vi "RRI_FFT.vi"() -> ()   [LabVIEW 2023]
uses:
  <vilib>/Analysis/4window.llb/windowTd.ctl
  <vilib>/measure/maspectr.llb/Power Spectrum and PSD Export Mode.ctl
  <vilib>/Analysis/2dsp.llb/Real FFT.vi
  <vilib>/measure/maspectr.llb/FFT Power Spectrum and PSD for 1 Chan (CDB).vi
  <vilib>/Utility/file.llb/Read Delimited Spreadsheet (DBL).vi
  <vilib>/gmath/NI_Gmath.lvlib
  <vilib>/Analysis/NI_AALPro.lvlib
  <vilib>/measure/NI_MAPro.lvlib
panel:
  out "LF/HF":dbl
  out "total power":dbl
  out "HF":dbl
  out "f0":dbl
  out "LF":dbl
  out "magnitude":dbl[](array[numeric])
  out "RRI baseline":cluster{"f0":dbl, "df":dbl, "magnitude":dbl[]}(graph)
  out "Power Spectrum / PSD":cluster{"f0":dbl, "df":dbl, "magnitude":dbl[]} {"magnitude" format="%.2p"; "f0" format="%0.2p"; "df" format="%0.2p"}
  out "baseline RRI inter":cluster{"xi used":dbl[], "yi":dbl[]}[](graph)
  out "RRI baseline 2":dbl[](graph)
  out "CW_baseline_index":dbl[](array[numeric])
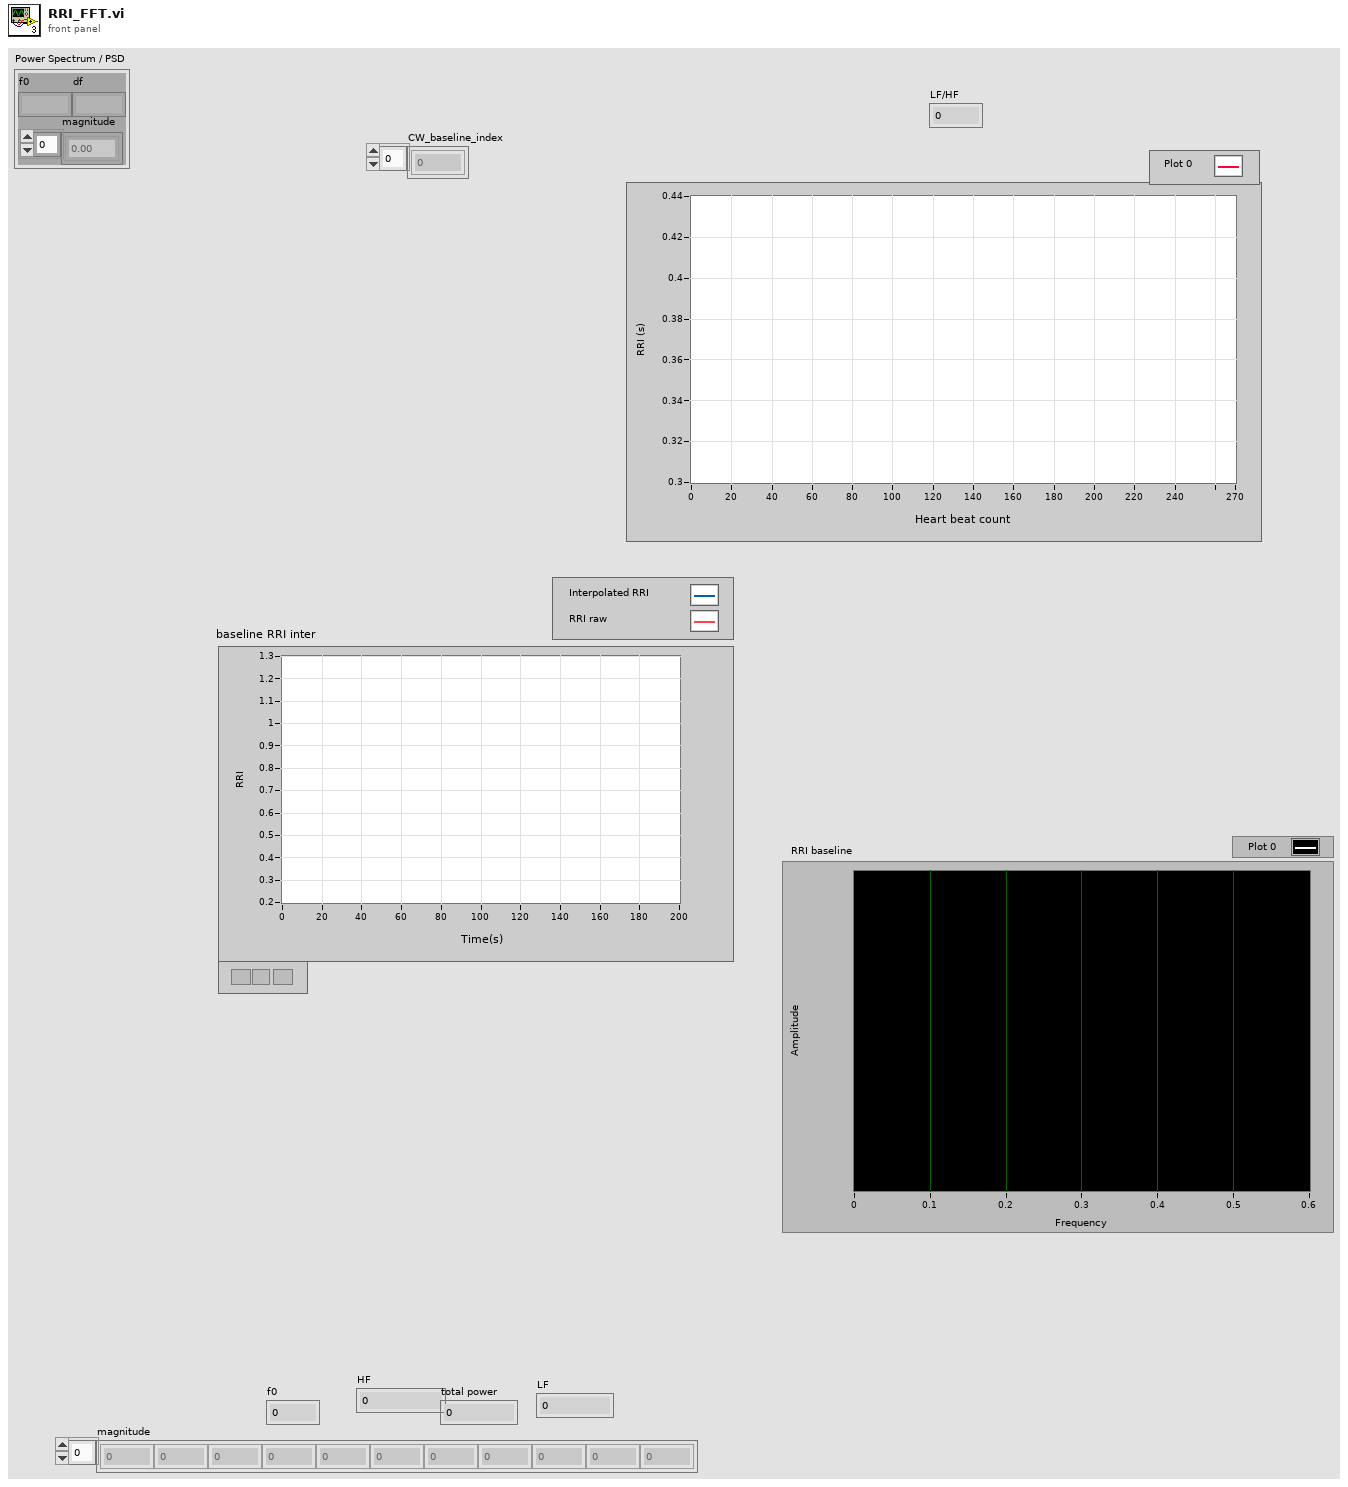
[diagram p1: front panel]
types:
  T1 = typedef "NI_MAPro.lvlib/Power Spectrum and PSD Export Mode.ctl" = u16
  T2 = typedef "NI_AALPro.lvlib/windowTd.ctl" = u32
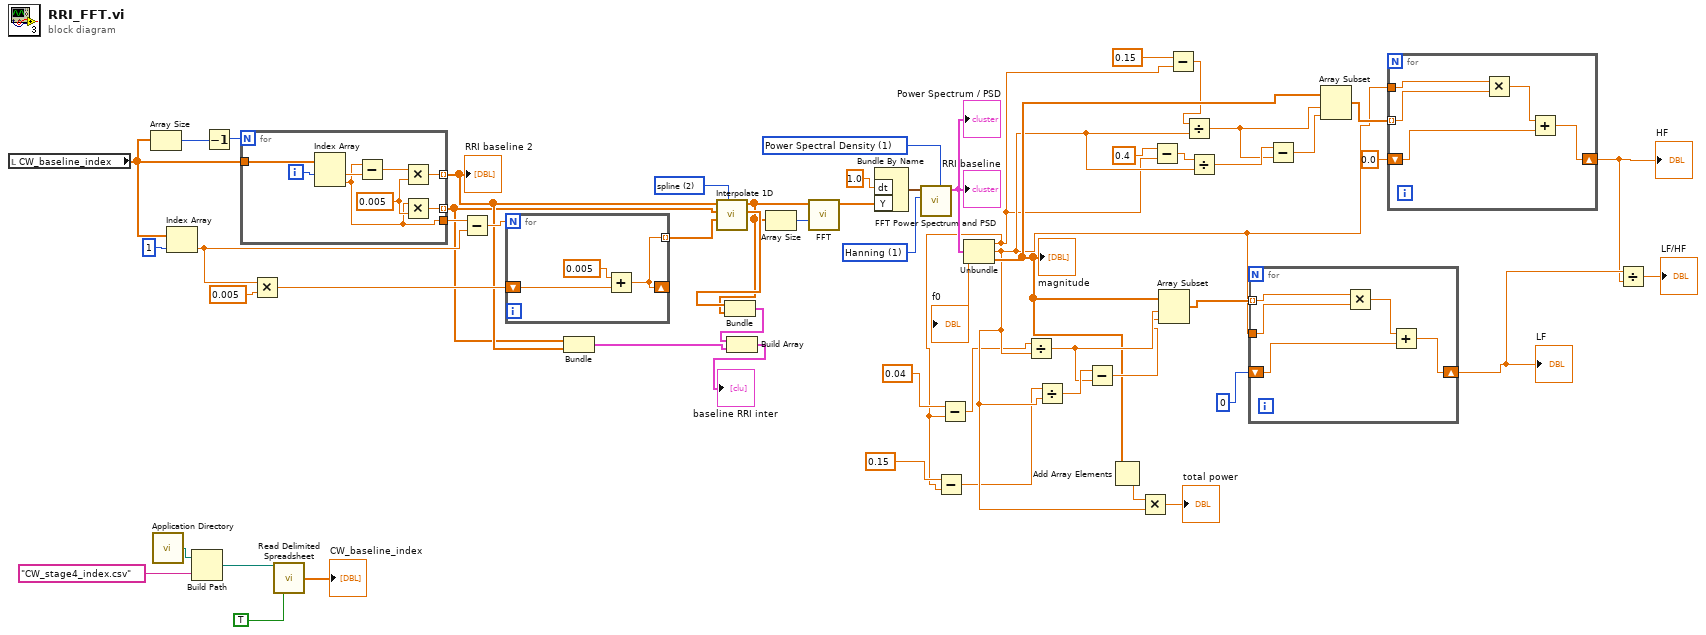
[diagram p0: block diagram]
diagram:
  w34 = T1 1 items=["Power Spectrum", "Power Spectral Density"] ("export mode")
  w35 = T2 1 items=["Rectangle"=0, "Hanning"=1, "Hamming"=2, "Blackman-Harris"=3, "Exact Blackman"=4, "Blackman"=5, "Flat Top"=6, "4 Term B-Harris "=7, "7 Term B-Harris"=8, "Low Sidelobe"=9, "Blackman Nuttall"=11, "Triangle"=30, "Bartlett-Hanning"=31, "Bohman"=32, "Parzen"=33, "Welch"=34, "Kaiser"=60, "Dolph-Chebyshev"=61, "Gaussian"=62] ("window")
  w54 = 2 items=["nearest", "linear", "spline", "cubic Hermite", "Lagrange"] ("method")
  n1 = local read "CW_baseline_index"() -> (w43:dbl[])
  n2 = Array Size(array=w43) -> (size(s)=w56:i32)
  n3 = call <vilib>:"Application Directory.vi"() -> ("Application Directory"=w31:path)
  n4 = Index Array(array=w43, index=1) -> (element=w51:dbl)
  n5 = Build Path(base path=w31, name or relative path="CW_stage4_index.csv") -> (appended path=w28:path)
  n6 = Decrement(x=w56) -> (x-1=w55:i32)
  n7 = for {
    N: w55 -> [_]
    tunnel: w43 -> [w64]
    tunnel: [w61] -> w47 mode=indexing
    tunnel: [w58] -> w45 mode=indexing
    tunnel: [w57] -> w52
    i -> [w63]
    w59 = 0.005 ("y")
    n8 = Index Array(array=w64, index #1=w63) -> (element #1=w62:dbl, element #2=w57:dbl)  [unwired: 1 in]
    n9 = Subtract(x=w57, y=w62) -> (x-y=w60:dbl)
    n10 = Multiply(x=w60, y=w59) -> (x*y=w61:dbl)
    n11 = Multiply(x=w57, y=w59) -> (x*y=w58:dbl)
  }
  "RRI baseline 2" <- w47
  n12 = Multiply(x=w51, y=0.005) -> (x*y=w49:dbl)
  n13 = call-poly <vilib>:"Read Delimited Spreadsheet.vi"("file path (dialog if empty)"=w28, "transpose? (F)"=TRUE) -> ("first row"=→"CW_baseline_index":dbl[])  [unwired: 8 in, 5 out]
  n14 = Subtract(x=w52, y=w51) -> (x-y=w48:dbl)
  n15 = for {
    N: w48 -> [_]
    shift-right: [w66] -> _
    shift-left: w49 -> [w67]
    tunnel: [w66] -> w44 mode=indexing
    n16 = Add(x=0.005 ("y"), y=w67) -> (x+y=w66:dbl)
  }
  n17 = Bundle(w45, w47) -> (w46:cluster{dbl[], dbl[]})  [unwired: 1 in]
  n18 = call <vilib>:"Interpolate 1D.vi"("method"=w54, "xi"=w44, "X"=w45, "Y"=w47) -> ("xi used"=w41:dbl[], "yi"=w32:dbl[])  [unwired: 5 in, 1 out]
  n19 = Bundle("xi used"=w41, "yi"=w32) -> (w40:cluster{"xi used":dbl[], "yi":dbl[]})  [unwired: 1 in]
  n20 = Build Array(w40, w46) -> (→"baseline RRI inter":cluster{"xi used":dbl[], "yi":dbl[]}[])
  n21 = Array Size(array=w32) -> (size(s)=w39:i32)
  n22 = call-poly <vilib>:"FFT.vi"("FFT size"=w39, "X"=w32) -> ("FFT {X}"=w37:cdb[])  [unwired: 8 in, 1 out]
  n23 = Bundle By Name("dt"=1.0, "Y"=w37) -> (w36:waveform(cdb))  [unwired: 1 in]
  n24 = call-poly <vilib>:"FFT Power Spectrum and PSD.vi"("export mode"=w34, "window"=w35, "time signal"=w36) -> ("Power Spectrum / PSD"=w33:cluster{"f0":dbl, "df":dbl, "magnitude":dbl[]})  [unwired: 5 in, 3 out]
  "Power Spectrum / PSD" <- w33
  "RRI baseline" <- w33
  n25 = Unbundle(w33) -> ("f0"=w5:dbl, "df"=w14:dbl, "magnitude"=w16:dbl[])
  "magnitude" <- w16
  "f0" <- w5
  n26 = Subtract(x=0.15, y=w5) -> (x-y=w9:dbl)
  n27 = Subtract(x=0.04, y=w5) -> (x-y=w11:dbl)
  n28 = Divide(x=w11, y=w14) -> (x/y=w25:dbl)
  n29 = Divide(x=w9, y=w14) -> (x/y=w26:dbl)
  n30 = Subtract(x=w26, y=w25) -> (x-y=w24:dbl)
  n31 = Add Array Elements(numeric array=w16) -> (sum=w15:dbl)
  n32 = Multiply(x=w15, y=w14) -> (x*y=→"total power":dbl)
  n33 = Subtract(x=0.4, y=w5) -> (x-y=w6:dbl)
  n34 = Array Subset(array=w16, index=w25, length=w24) -> (w22:dbl[])
  n35 = Subtract(x=0.15, y=w5) -> (x-y=w7:dbl)
  n36 = Divide(x=w7, y=w14) -> (x/y=w20:dbl)
  n37 = Divide(x=w6, y=w14) -> (x/y=w21:dbl)
  n38 = for {
    shift-right: [w68] -> w3
    shift-left: 0 -> [w69]
    tunnel: w22 -> [w71] mode=indexing
    tunnel: w14 -> [w72]
    n39 = Multiply(x=w71, y=w72) -> (x*y=w70:dbl)
    n40 = Add(x=w70, y=w69) -> (x+y=w68:dbl)
  }
  "LF" <- w3
  n41 = Subtract(x=w21, y=w20) -> (x-y=w19:dbl)
  n42 = Array Subset(array=w16, index=w20, length=w19) -> (w18:dbl[])
  n43 = for {
    shift-right: [w73] -> w2
    shift-left: 0.0 -> [w74]
    tunnel: w14 -> [w76]
    tunnel: w18 -> [w77] mode=indexing
    n44 = Multiply(x=w76, y=w77) -> (x*y=w75:dbl)
    n45 = Add(x=w75, y=w74) -> (x+y=w73:dbl)
  }
  "HF" <- w2
  n46 = Divide(x=w3, y=w2) -> (x/y=→"LF/HF":dbl)
